vi "HTML_Table_Head.vi"(8 "entrée d'erreur (pas d'erreur)":errorcluster caption="errin", 10 "Tableau":string[](array[string]), 11 "chaîne en entrée":string) -> (0 "sortie d'erreur":errorcluster caption="errout", 3 "result string":string)   [LabVIEW 2017]
doc: "permets de creer l'entete"
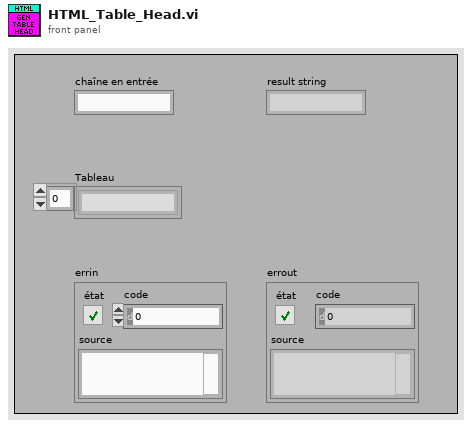
[diagram p1: front panel]
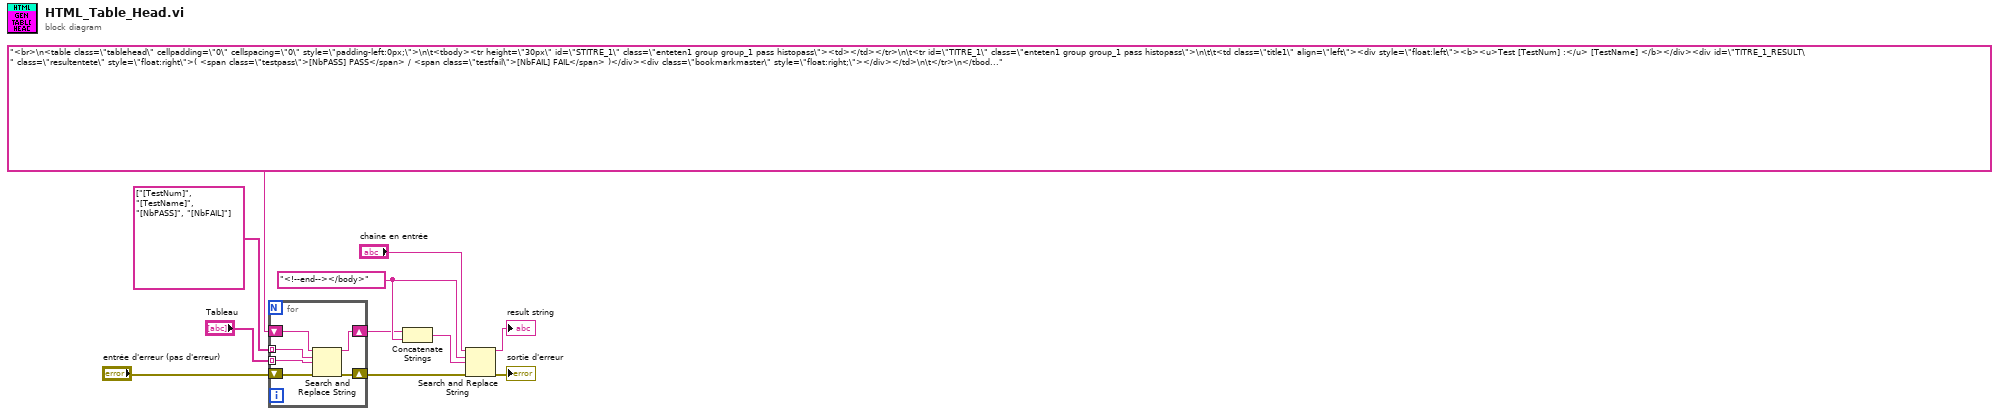
[diagram p0: block diagram]
diagram:
  w8 = "<!--end--></body>" ("chaîne recherchée")
  n1 = for {
    tunnel: string[] ["[TestNum]", "[TestName]", "[NbPASS]", "[NbFAIL]"] -> [w16] mode=indexing
    tunnel: "Tableau" -> [w15] mode=indexing
    shift-right: [w13] -> w9
    shift-left: "entrée d'erreur (pas d'erreur)" -> [w14]
    shift-right: [w12] -> w7
    shift-left: "<br>\n<table class=\"tablehead\" cellpadding=\"0\" cellspacing=\"0\" style=\"padding-left:0px;\">\n\t<tbody><tr height=\"30px\" id=\"STITRE_1\" class=\"enteten1 group group_1 pass histopass\"><td></td></tr>\n\t<tr id=\"TITRE_1\" class=\"enteten1 group group_1 pass histopass\">\n\t\t<td class=\"title1\" align=\"left\"><div style=\"float:left\"><b><u>Test [TestNum] :</u> [TestName] </b></div><div id=\"TITRE_1_RESULT\" class=\"resultentete\" style=\"float:right\">( <span class=\"testpass\">[NbPASS] PASS</span> / <span class=\"testfail\">[NbFAIL] FAIL</span> )</div><div class=\"bookmarkmaster\" style=\"float:right;\"></div></td>\n\t</tr>\n</tbody></table>" -> [w17]
    n2 = Search and Replace String(input string=w17, search string=w16, replace string=w15, error in=w14) -> (result string=w12:string, error out=w13:errorcluster)  [unwired: 4 in, 2 out]
  }
  n3 = Concatenate Strings(w7, w8) -> (w6:string)
  n4 = Search and Replace String(input string="chaîne en entrée", search string=w8, replace string=w6, error in=w9) -> (result string=→"result string":string, error out=→"sortie d'erreur":errorcluster)  [unwired: 4 in, 2 out]
